vi "ExCameraNadvdisp.vi"() -> ()   [LabVIEW 2010]
uses:
  Open-Close/CamHandle.vi
panel:
  in  "done flag":bool
  in  "Exposure":dbl=0.01 min=0.0 step=0.01 format="%.2f"
  out "error out":errorcluster
  in  "error in (no error)":errorcluster
  in  "SITKFULLDISPLAYLib.SITKFullDisplay":refnum<k7>(container)
  # "NOTICE\n\nTHIS VI USES A GLOBAL CAMERA HANDLE\n\nTHE VI EXOPENGLOBALCAM.VI MUST BE\nRUN AT THE START OF THE WORK SESSION.\nTHE CAMERA WILL REMAIN OPENED.\n\nTHE VI EXCLOSEGLOBALCAM.VI MUST\nBE RUN BEFORE LEAVING LABVIEW."
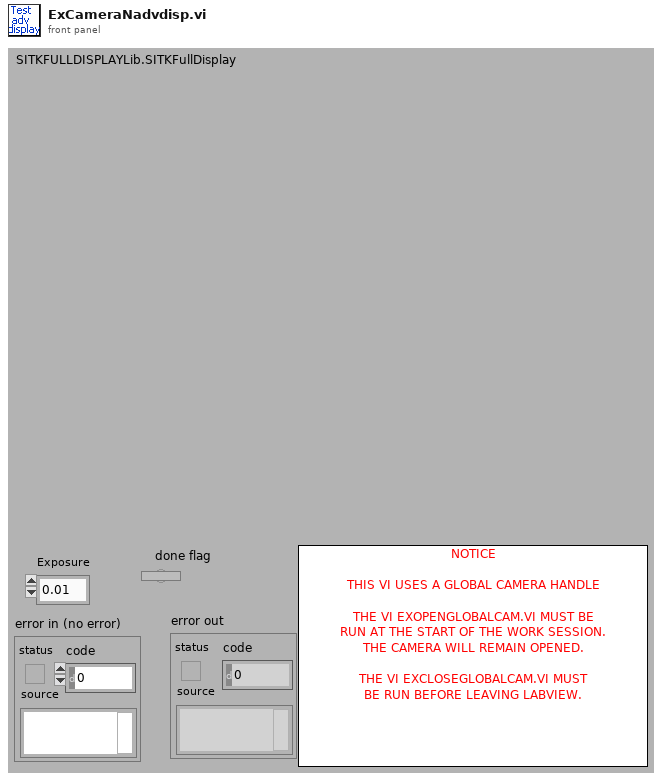
[diagram p1: front panel]
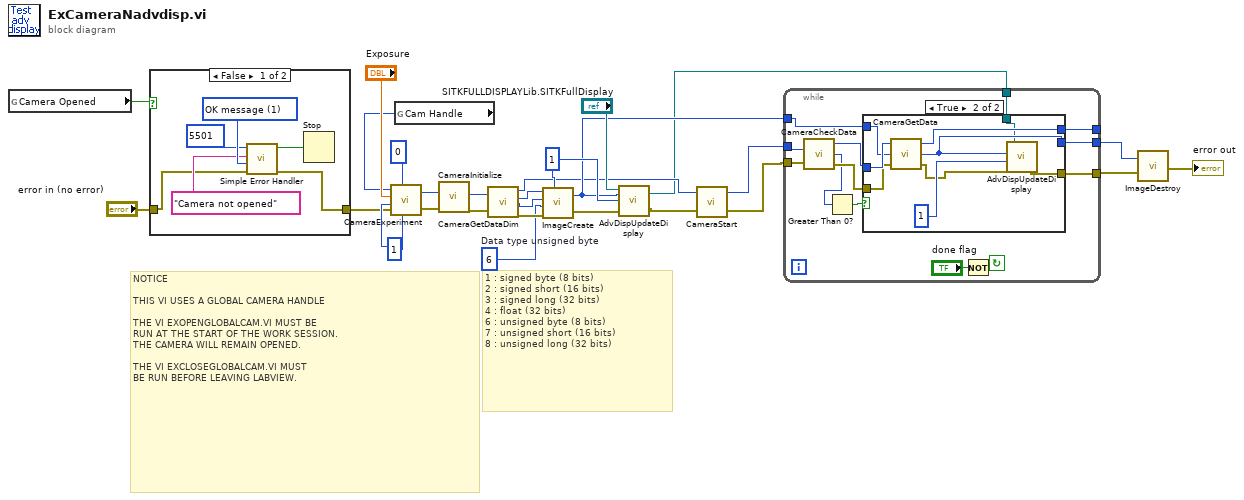
[diagram p0: block diagram]
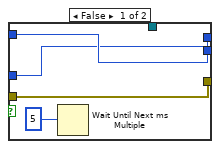
[diagram p3: hidden frame]
diagram:
  w15 = 6  # Data type unsigned byte
  w24 = 1
  w27 = 1
  # "NOTICE\n\nTHIS VI USES A GLOBAL CAMERA HANDLE\n\nTHE VI EXOPENGLOBALCAM.VI MUST BE\nRUN AT THE START OF THE WORK SESSION.\nTHE CAMERA WILL REMAIN OPENED.\n\nTHE VI EXCLOSEGLOBALCAM.VI MUST\nBE RUN BEFORE LEAVING LABVIEW."
  # "1 : signed byte (8 bits)\n2 : signed short (16 bits)\n3 : signed long (32 bits)\n4 : float (32 bits)\n6 : unsigned byte (8 bits)\n7 : unsigned short (16 bits)\n8 : unsigned long (32 bits)"
  n1 = global read "CamHandle.vi" "Camera Opened"() -> (w4:bool)
  n2 = case shown="False" w4 {
    tunnel: "error in (no error)" -> [w29 w34]
    tunnel: [w28 w34] -> w5
    frame False {
      w33 = u16 1 items=["no dialog", "OK message", "continue or stop message"] ("type of dialog (OK msg:1)")
      n3 = call <vilib>:"Simple Error Handler.vi"("error code (no error:0)"=5501, "error source (\" \")"="Camera not opened", "type of dialog (OK msg:1)"=w33, "error in (no error)"=w29) -> ("error?"=w31:bool, "error out"=w28:errorcluster)  [unwired: 1 in, 3 out]
      n4 = Stop(stop? (T)=w31) -> ()
    }
    frame True {
    }
  }
  n5 = global read "CamHandle.vi" "Cam Handle"() -> (w3:u32)
  n6 = call <userlib>:"CameraExperiment.vi"("Number of Accumulations"=w24, "Acquire / Focus Flag"=0, "error in"=w5, "Number of Images"=w24, "Exposure (sec)"="Exposure", "Camera Handle"=w3) -> ("error out"=w22:errorcluster, "Camera Handle"=w21:u32)
  n7 = call <userlib>:"CameraInitialize.vi"("error in"=w22, "Camera Handle"=w21) -> ("error out"=w20:errorcluster, "Camera Handle"=w19:u32)
  n8 = call <userlib>:"CameraGetDataDim.vi"("Camera Handle"=w19, "error in"=w20) -> ("Camera Handle"=w11:u32, "Xdim"=w17:u32, "Ydim"=w16:u32, "error out"=w18:errorcluster)
  n9 = call <userlib>:"ImageCreate.vi"("X dimension"=w17, "Y dimension"=w16, "Data Type"=w15, "error in"=w18, "Number Of Frames"=w27) -> ("Image Handle"=w14:u32, "error out"=w13:errorcluster)
  n10 = call <userlib>:"AdvDispUpdateDisplay.vi"("error in (no error)"=w13, "Frame Number To Display"=w27, "Image Handle"=w14, "SITKFULLDISPLAYLib.SITKFullDisplay"="SITKFULLDISPLAYLib.SITKFullDisplay") -> ("error out"=w12:errorcluster, "SITKFULLDISPLAYLib.SITKFullDisplay"=w7:refnum<k7>)
  n11 = call <userlib>:"CameraStart.vi"("error in"=w12, "Camera Handle"=w11) -> ("error out"=w9:errorcluster, "Camera Handle"=w10:u32)
  n12 = while {
    tunnel: w10 -> [w40]
    tunnel: w9 -> [w39]
    tunnel: [w43] -> w2
    tunnel: [w42] -> w8
    tunnel: [w47] -> _
    tunnel: w14 -> [w46]
    tunnel: w7 -> [w35]
    stop <- w44 continue-if-true
    n13 = call <userlib>:"CameraCheckData.vi"("Camera Handle"=w40, "error in"=w39) -> ("Camera Handle"=w38:u32, "Number Of Frames Available"=w36:i32, "error out"=w41:errorcluster)
    n14 = Greater Than 0?(x=w36) -> (x > 0?=w37:bool)
    n15 = case shown="True" w37 {
      tunnel: w38 -> [w49 w60]
      tunnel: w41 -> [w51 w59]
      tunnel: [w49 w58] -> w47
      tunnel: w46 -> [w50 w57]
      tunnel: [w51 w53] -> w43
      tunnel: [w50 w56] -> w42
      tunnel: w35 -> [_ w52]
      frame False {
        n16 = Wait Until Next ms Multiple(millisecond multiple=5) -> ()  [unwired: 1 out]
      }
      frame True {
        n17 = call <userlib>:"CameraGetData.vi"("error in"=w59, "Data Handle"=w57, "Camera Handle"=w60) -> ("error out"=w54:errorcluster, "Data Handle"=w56:u32, "Camera Handle"=w58:u32)
        n18 = call <userlib>:"AdvDispUpdateDisplay.vi"("error in (no error)"=w54, "Frame Number To Display"=1, "Image Handle"=w56, "SITKFULLDISPLAYLib.SITKFullDisplay"=w52) -> ("error out"=w53:errorcluster)  [unwired: 1 out]
      }
    }
    n19 = Not(x="done flag") -> (.not. x?=w44:bool)
  }
  n20 = call <userlib>:"ImageDestroy.vi"("error in"=w2, "Data handle"=w8) -> ("error out"=→"error out":errorcluster)
